vi "CG_sub.vi"() -> ()   [LabVIEW 2018]
uses:
  <vilib>/Instr/_visa.llb/VISA Configure Serial Port (Instr).vi
panel:
  out "Расстояние на \nускорение [мм]":dbl
  out "Концевики":u16(ring) items=["Выкл", "Вкл"]
  in  "Концевик":bool
  in  "Стоп":bool
  in  "Axis":bool
  in  "Direction":bool
  in  "смещение":bool
  out "Смещение [имп]":dbl
  in  "Смещение[мм]":dbl
  in  "Хоуминг Y":bool
  in  "Хоуминг X":bool
  in  "COM port":refnum<visa-resource-name>
  out "Скорость [имп/сек]":dbl
  out "Ширинм [имп]":dbl
  in  "Скорость [мм/сек]":dbl
  out "Высота [имп]":dbl
  in  "Коэфициент пересчета [1/мм]":dbl
  in  "Записать":bool
  in  "Число повторений":dbl
  in  "Ширина [мм]":dbl
  in  "Высота [мм]":dbl
  in  "Время разгона/торможения [мс]":dbl
  in  "Close":bool
  # "Ручной режим"
  # "Автоматический режим"
  # ".\n.\n."
  # "Y"
  # "X"
  # "pos"
  # "Neg"
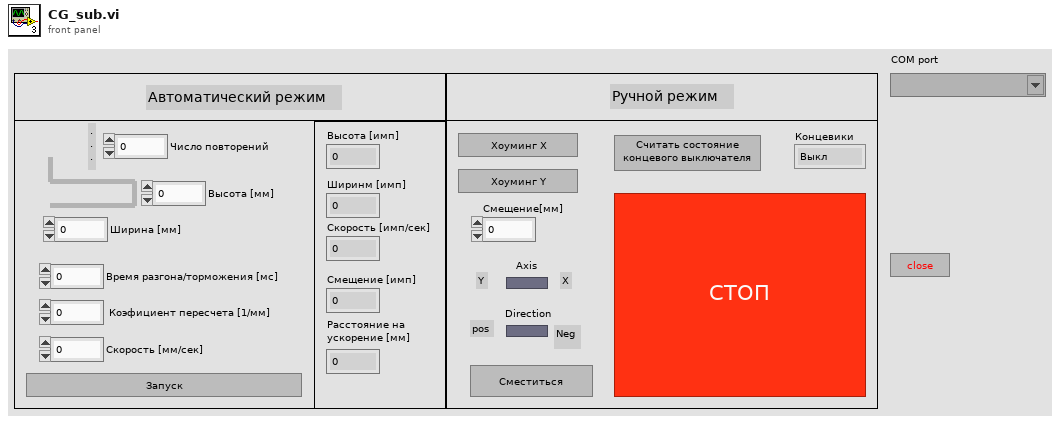
[diagram p1: front panel]
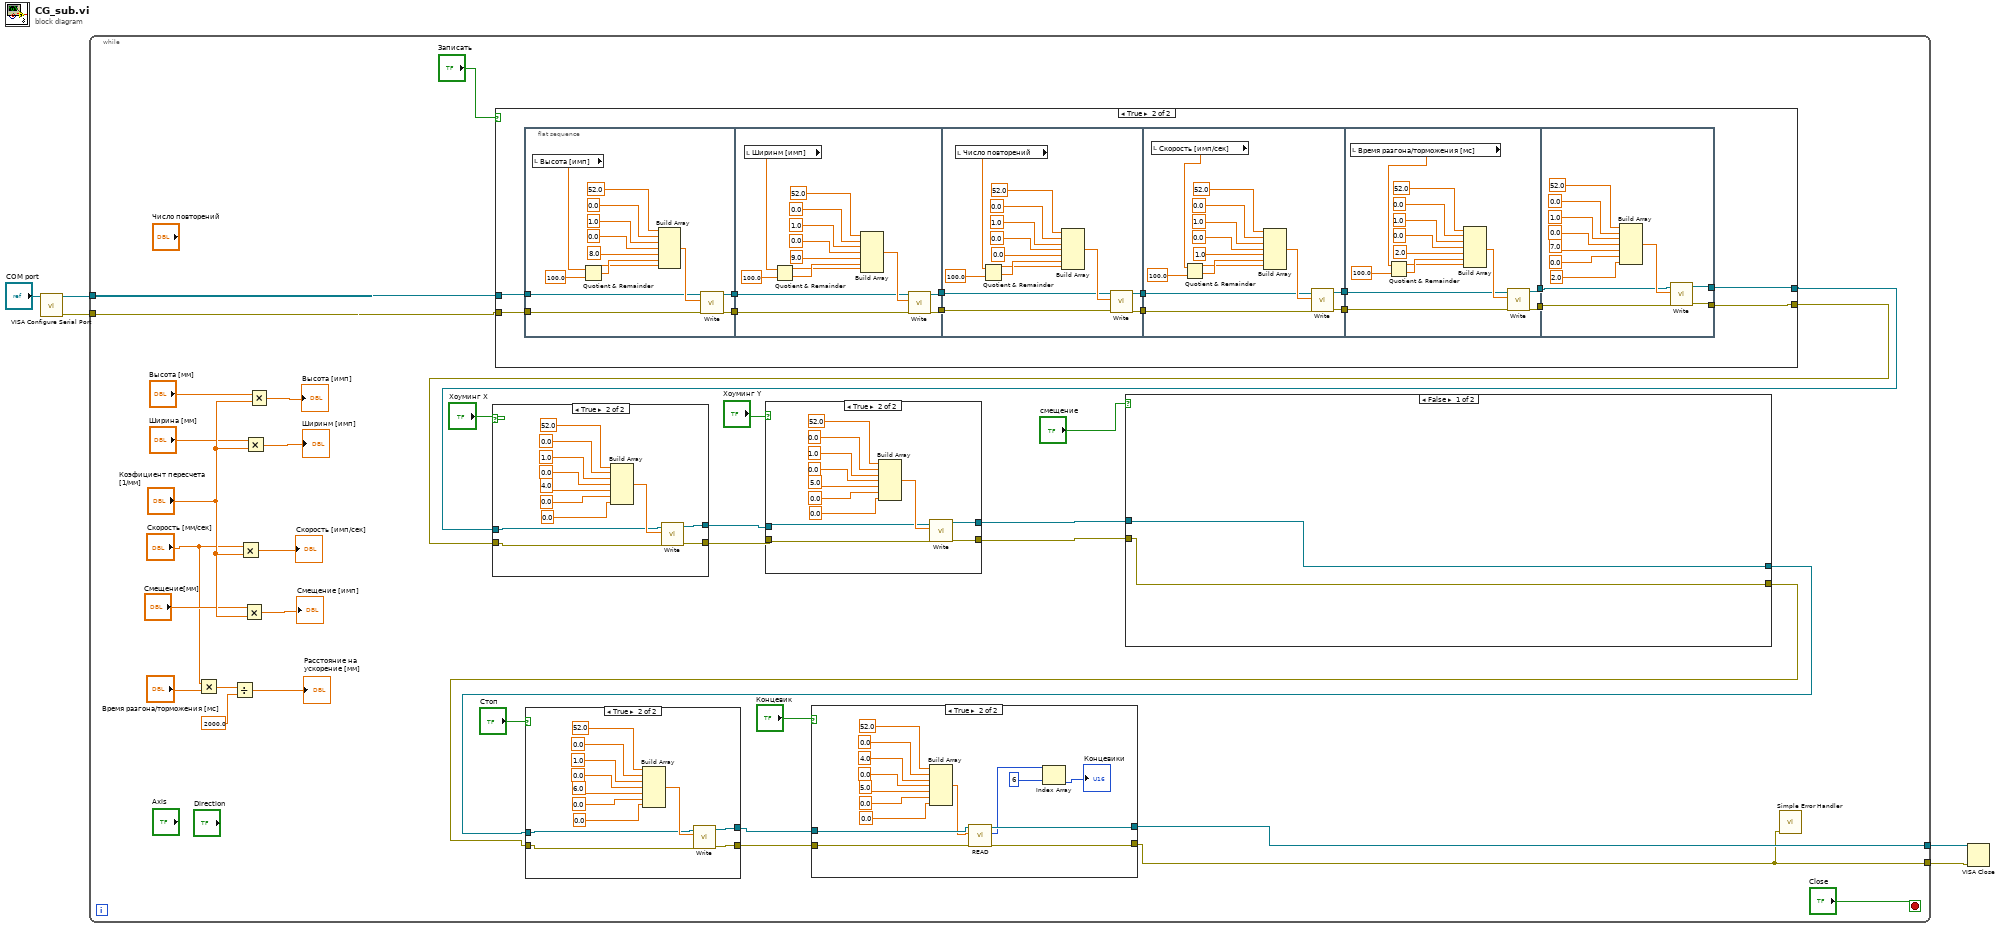
[diagram p0: block diagram]
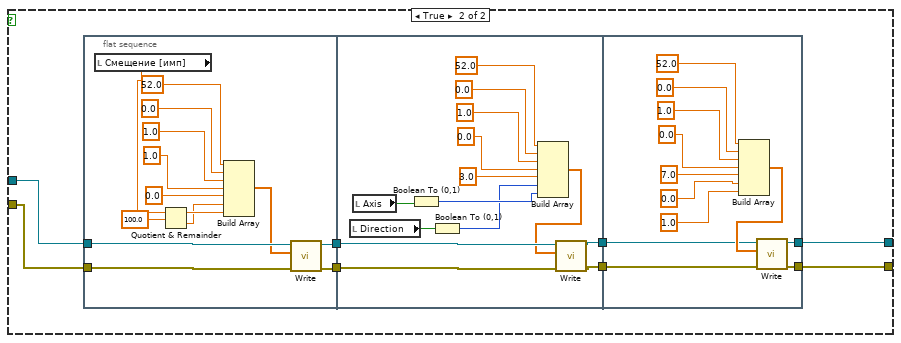
[diagram p4: hidden frame]
diagram:
  n1 = call-poly "VISA Configure Serial Port"("VISA resource name"="COM port") -> ("VISA resource name out"=w4:refnum<visa-resource-name>, "error out"=w3:errorcluster)  [unwired: 13 in]
  n2 = while {
    tunnel: w4 -> [w37]
    tunnel: w3 -> [w36]
    tunnel: [w11] -> w2
    tunnel: [w12] -> w1
    stop <- "Close" stop-if-true
    n3 = Multiply(x="Скорость [мм/сек]", y="Время разгона/торможения [мс]") -> (x*y=w10:dbl)
    n4 = Divide(x=w10, y=2000.0) -> (x/y=→"Расстояние на \nускорение [мм]":dbl)
    n5 = Multiply(x="Скорость [мм/сек]", y="Коэфициент пересчета [1/мм]") -> (x*y=→"Скорость [имп/сек]":dbl)
    n6 = Multiply(x="Смещение[мм]", y="Коэфициент пересчета [1/мм]") -> (x*y=→"Смещение [имп]":dbl)
    n7 = Multiply(x="Ширина [мм]", y="Коэфициент пересчета [1/мм]") -> (x*y=→"Ширинм [имп]":dbl)
    n8 = Multiply(x="Высота [мм]", y="Коэфициент пересчета [1/мм]") -> (x*y=→"Высота [имп]":dbl)
    n9 = case shown="True" "Записать" {
      tunnel: w37 -> [w150 w164]
      tunnel: w36 -> [w149 w163]
      tunnel: [w150 w152] -> w33
      tunnel: [w149 w151] -> w34
      frame False {
      }
      frame True {
        n10 = flat-sequence {
          tunnel: w164 -> [w168]
          tunnel: w163 -> [w167]
          tunnel: [w166] -> w162
          tunnel: [w165] -> w161
          tunnel: w162 -> [w180]
          tunnel: w161 -> [w179]
          tunnel: [w182] -> w160
          tunnel: [w181] -> w159
          tunnel: w160 -> [w197]
          tunnel: w159 -> [w196]
          tunnel: [w195] -> w158
          tunnel: [w194] -> w157
          tunnel: w158 -> [w211]
          tunnel: w157 -> [w210]
          tunnel: [w208] -> w156
          tunnel: [w207] -> w155
          tunnel: w156 -> [w224]
          tunnel: w155 -> [w223]
          tunnel: [w225] -> w154
          tunnel: [w221] -> w153
          tunnel: w154 -> [w236]
          tunnel: w153 -> [w235]
          tunnel: [w240] -> w152
          tunnel: [w239] -> w151
          frame #0 {
            n11 = local read "Высота [имп]"() -> (w177:dbl)
            n12 = Quotient & Remainder(x=w177, y=100.0) -> (x-y*floor(x/y)=w170:dbl, floor(x/y)=w171:dbl)
            n13 = Build Array(52.0 ("element"), 0.0 ("element"), 1.0 ("element"), 0.0 ("element"), 8.0 ("element"), w171, w170) -> (w169:dbl[])
            n14 = call "Write.vi"("VISA resource name"=w168, "unsigned byte array"=w169, "error in (no error)"=w167) -> ("VISA resource name out"=w166:refnum<visa-resource-name>, "error out"=w165:errorcluster)  [unwired: 4 in]
          }
          frame #1 {
            n15 = local read "Ширинм [имп]"() -> (w183:dbl)
            n16 = Quotient & Remainder(x=w183, y=100.0) -> (x-y*floor(x/y)=w185:dbl, floor(x/y)=w186:dbl)
            n17 = Build Array(52.0 ("element"), 0.0 ("element"), 1.0 ("element"), 0.0 ("element"), 9.0 ("element"), w186, w185) -> (w184:dbl[])
            n18 = call "Write.vi"("VISA resource name"=w180, "unsigned byte array"=w184, "error in (no error)"=w179) -> ("VISA resource name out"=w182:refnum<visa-resource-name>, "error out"=w181:errorcluster)  [unwired: 4 in]
          }
          frame #2 {
            n19 = local read "Число повторений"() -> (w193:dbl)
            n20 = Quotient & Remainder(x=w193, y=100.0) -> (x-y*floor(x/y)=w199:dbl, floor(x/y)=w200:dbl)
            n21 = Build Array(52.0 ("element"), 0.0 ("element"), 1.0 ("element"), 0.0 ("element"), 0.0 ("element"), w200, w199) -> (w198:dbl[])
            n22 = call "Write.vi"("VISA resource name"=w197, "unsigned byte array"=w198, "error in (no error)"=w196) -> ("VISA resource name out"=w195:refnum<visa-resource-name>, "error out"=w194:errorcluster)  [unwired: 4 in]
          }
          frame #3 {
            n23 = local read "Скорость [имп/сек]"() -> (w209:dbl)
            n24 = Quotient & Remainder(x=w209, y=100.0) -> (x-y*floor(x/y)=w213:dbl, floor(x/y)=w214:dbl)
            n25 = Build Array(52.0 ("element"), 0.0 ("element"), 1.0 ("element"), 0.0 ("element"), 1.0 ("element"), w214, w213) -> (w212:dbl[])
            n26 = call "Write.vi"("VISA resource name"=w211, "unsigned byte array"=w212, "error in (no error)"=w210) -> ("VISA resource name out"=w208:refnum<visa-resource-name>, "error out"=w207:errorcluster)  [unwired: 4 in]
          }
          frame #4 {
            n27 = local read "Время разгона/торможения [мс]"() -> (w222:dbl)
            n28 = Quotient & Remainder(x=w222, y=100.0) -> (x-y*floor(x/y)=w227:dbl, floor(x/y)=w228:dbl)
            n29 = Build Array(52.0 ("element"), 0.0 ("element"), 1.0 ("element"), 0.0 ("element"), 2.0 ("element"), w228, w227) -> (w226:dbl[])
            n30 = call "Write.vi"("VISA resource name"=w224, "unsigned byte array"=w226, "error in (no error)"=w223) -> ("VISA resource name out"=w225:refnum<visa-resource-name>, "error out"=w221:errorcluster)  [unwired: 4 in]
          }
          frame #5 {
            n31 = Build Array(52.0 ("element"), 0.0 ("element"), 1.0 ("element"), 0.0 ("element"), 7.0 ("element"), 0.0 ("element"), 2.0 ("element")) -> (w241:dbl[])
            n32 = call "Write.vi"("VISA resource name"=w236, "unsigned byte array"=w241, "error in (no error)"=w235) -> ("VISA resource name out"=w240:refnum<visa-resource-name>, "error out"=w239:errorcluster)  [unwired: 4 in]
          }
        }
      }
    }
    n33 = case shown="True" "Хоуминг X" {
      tunnel: w34 -> [w135 w139]
      tunnel: w33 -> [w136 w140]
      tunnel: [w136 w138] -> w31
      tunnel: [w135 w137] -> w30
      frame False {
      }
      frame True {
        n34 = Build Array(52.0 ("element"), 0.0 ("element"), 1.0 ("element"), 0.0 ("element"), 4.0 ("element"), 0.0 ("element"), 0.0 ("element")) -> (w143:dbl[])
        n35 = call "Write.vi"("VISA resource name"=w140, "unsigned byte array"=w143, "error in (no error)"=w139) -> ("VISA resource name out"=w138:refnum<visa-resource-name>, "error out"=w137:errorcluster)  [unwired: 4 in]
      }
    }
    n36 = case shown="True" "Хоуминг Y" {
      tunnel: w30 -> [w121 w125]
      tunnel: w31 -> [w122 w126]
      tunnel: [w122 w124] -> w29
      tunnel: [w121 w123] -> w28
      frame False {
      }
      frame True {
        n37 = Build Array(52.0 ("element"), 0.0 ("element"), 1.0 ("element"), 0.0 ("element"), 5.0 ("element"), 0.0 ("element"), 0.0 ("element")) -> (w129:dbl[])
        n38 = call "Write.vi"("VISA resource name"=w126, "unsigned byte array"=w129, "error in (no error)"=w125) -> ("VISA resource name out"=w124:refnum<visa-resource-name>, "error out"=w123:errorcluster)  [unwired: 4 in]
      }
    }
    n39 = case shown="False" "смещение" {
      tunnel: w29 -> [w72 w80]
      tunnel: w28 -> [w71 w79]
      tunnel: [w72 w74] -> w17
      tunnel: [w71 w73] -> w16
      frame False {
      }
      frame True {
        n40 = flat-sequence {
          tunnel: w80 -> [w92]
          tunnel: w79 -> [w91]
          tunnel: [w90] -> w78
          tunnel: [w89] -> w77
          tunnel: w78 -> [w108]
          tunnel: w77 -> [w107]
          tunnel: [w96] -> w76
          tunnel: [w95] -> w75
          tunnel: w76 -> [w114]
          tunnel: w75 -> [w113]
          tunnel: [w110] -> w74
          tunnel: [w109] -> w73
          frame #0 {
            n41 = local read "Смещение [имп]"() -> (w94:dbl)
            n42 = Quotient & Remainder(x=w94, y=100.0) -> (x-y*floor(x/y)=w87:dbl, floor(x/y)=w86:dbl)
            n43 = Build Array(52.0 ("element"), 0.0 ("element"), 1.0 ("element"), 1.0 ("element"), 0.0 ("element"), w86, w87) -> (w88:dbl[])
            n44 = call "Write.vi"("VISA resource name"=w92, "unsigned byte array"=w88, "error in (no error)"=w91) -> ("VISA resource name out"=w90:refnum<visa-resource-name>, "error out"=w89:errorcluster)  [unwired: 4 in]
          }
          frame #1 {
            n45 = local read "Direction"() -> (w105:bool)
            n46 = local read "Axis"() -> (w106:bool)
            n47 = Boolean To (0,1)(Boolean=w106) -> (0, 1=w98:i16)
            n48 = Boolean To (0,1)(Boolean=w105) -> (0, 1=w97:i16)
            n49 = Build Array(52.0 ("element"), 0.0 ("element"), 1.0 ("element"), 0.0 ("element"), 3.0 ("element"), w97, w98) -> (w99:dbl[])
            n50 = call "Write.vi"("VISA resource name"=w108, "unsigned byte array"=w99, "error in (no error)"=w107) -> ("VISA resource name out"=w96:refnum<visa-resource-name>, "error out"=w95:errorcluster)  [unwired: 4 in]
          }
          frame #2 {
            n51 = Build Array(52.0 ("element"), 0.0 ("element"), 1.0 ("element"), 0.0 ("element"), 7.0 ("element"), 0.0 ("element"), 1.0 ("element")) -> (w115:dbl[])
            n52 = call "Write.vi"("VISA resource name"=w114, "unsigned byte array"=w115, "error in (no error)"=w113) -> ("VISA resource name out"=w110:refnum<visa-resource-name>, "error out"=w109:errorcluster)  [unwired: 4 in]
          }
        }
      }
    }
    n53 = case shown="True" "Стоп" {
      tunnel: w16 -> [w57 w61]
      tunnel: w17 -> [w58 w62]
      tunnel: [w58 w60] -> w15
      tunnel: [w57 w59] -> w14
      frame False {
      }
      frame True {
        n54 = Build Array(52.0 ("element"), 0.0 ("element"), 1.0 ("element"), 0.0 ("element"), 6.0 ("element"), 0.0 ("element"), 0.0 ("element")) -> (w65:dbl[])
        n55 = call "Write.vi"("VISA resource name"=w62, "unsigned byte array"=w65, "error in (no error)"=w61) -> ("VISA resource name out"=w60:refnum<visa-resource-name>, "error out"=w59:errorcluster)  [unwired: 4 in]
      }
    }
    n56 = case shown="True" "Концевик" {
      tunnel: w15 -> [w40 w47]
      tunnel: [w40 w49] -> w12
      tunnel: [w41 w48] -> w11
      tunnel: w14 -> [w41 w46]
      frame False {
      }
      frame True {
        n57 = Build Array(52.0 ("element"), 0.0 ("element"), 4.0 ("element"), 0.0 ("element"), 5.0 ("element"), 0.0 ("element"), 0.0 ("element")) -> (w45:dbl[])
        n58 = call "READ.vi"("error in (no error)"=w46, "unsigned byte array 2"=w45, "VISA resource name"=w47) -> ("error out"=w48:errorcluster, "unsigned byte array"=w43:u8[], "VISA resource name out"=w49:refnum<visa-resource-name>)  [unwired: 6 in]
        n59 = Index Array(array=w43, index=u32 6 ("byte count")) -> (element=→"Концевики":u8)
      }
    }
    n60 = call <vilib>:"Simple Error Handler.vi"("error in (no error)"=w11) -> ()  [unwired: 1 in, 8 out]
  }
  n61 = VISA Close(VISA resource name=w1, error in (no error)=w2) -> ()  [unwired: 1 out]
